vi "Init.vi"(8 "error in (no error)":errorcluster, 10 "Name":string, 11 "Debug View In":refnum<class "Debug View.lvclass">) -> (0 "error out":errorcluster, 3 "Debug View Out":refnum<class "Debug View.lvclass">)   [LabVIEW 2020, in "Debug View.lvclass"]
doc: "Initializes the process and creates necessary references. Anything initialized here is released in the Clear.vi method."
uses:
  Debug View.lvclass
  Protected/Broadcasting/Broadcast Message Cluster.ctl
  Debug View.lvclass/Debug View.ctl
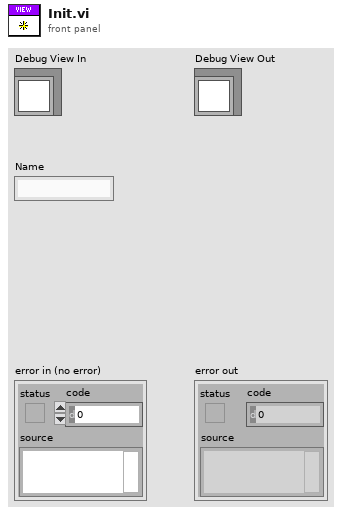
[diagram p1: front panel]
types:
  T1 = typedef "Debug View.lvclass/Broadcast Message Cluster.ctl" = cluster{"Sender":string, "Message":string, "Message Data":variant}
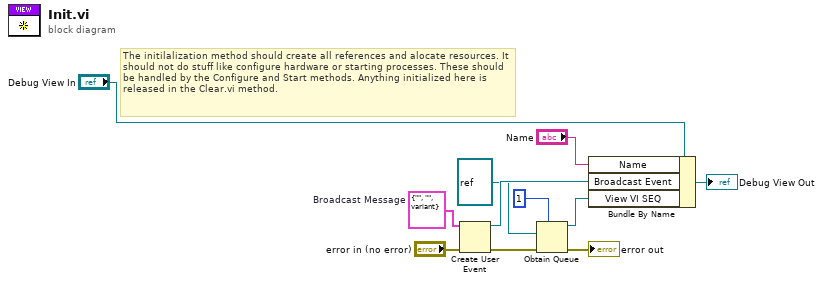
[diagram p0: block diagram]
diagram:
  w9 = T1 {"Sender"="", "Message"="", "Message Data"=variant}  # Broadcast Message
  # "The initilalization method should create all references and alocate resources. It should not do stuff like configure hardware or starting processes. These should be handled by the Configure and Start methods. Anything initialized here is released in the Clear.vi method."
  n1 = Create User Event(user event datatype=w9, error in="error in (no error)") -> (user event=w8:refnum<user-event>, error out=w4:errorcluster)
  n2 = Obtain Queue(max queue size (-1, unlimited)=1, element data type=refnum<vi> refnum ("This VI"), error in (no error)=w4) -> (queue out=w1:refnum<queue>, error out=→"error out":errorcluster)  [unwired: 2 in, 1 out]
  n3 = Bundle By Name(cluster="Debug View In", "Name"="Name", "Broadcast Event"=w8, "View VI SEQ"=w1) -> (→"Debug View Out":refnum<class "Debug View.lvclass">)
